vi "Angle To Angle Velocity.vi"(10 "Period":i64, 11 "Yaw":dbl) -> (3 "Yaw degrees/sec":dbl)   [LabVIEW 2014]
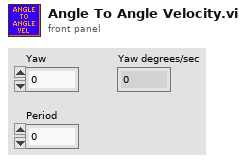
[diagram p1: front panel]
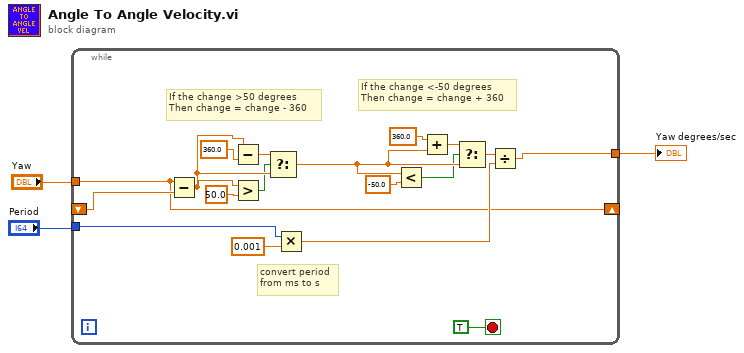
[diagram p0: block diagram]
diagram:
  n1 = while {
    tunnel: "Period" -> [w9]
    tunnel: [w5] -> w2
    shift-right: [w4] -> _
    shift-left: _ -> [w6]
    tunnel: "Yaw" -> [w4]
    stop <- TRUE stop-if-true
    # "convert period\nfrom ms to s"
    # "If the change <-50 degrees\nThen change = change + 360"
    # "If the change >50 degrees\nThen change = change - 360"
    n2 = Subtract(x=w4, y=w6) -> (x-y=w21:dbl)
    n3 = Subtract(x=w21, y=360.0) -> (x-y=w13:dbl)
    n4 = Greater?(x=w21, y=50.0) -> (0:w12:bool)
    n5 = Select(t=w13, s=w12, f=w21) -> (s? t:f=w18:dbl)
    n6 = Multiply(x=w9, y=0.001) -> (x*y=w10:dbl)
    n7 = Less?(x=w18, y=-50.0) -> (x < y?=w15:bool)
    n8 = Add(x=360.0 ("y"), y=w18) -> (x+y=w17:dbl)
    n9 = Select(t=w17, s=w15, f=w18) -> (s? t:f=w19:dbl)
    n10 = Divide(x=w19, y=w10) -> (x/y=w5:dbl)
  }
  "Yaw degrees/sec" <- w2
